vi "Read id.vi"(8 "error in (no error)":errorcluster, 11 "Motor in":refnum<class "Motor.lvclass">) -> (0 "error out":errorcluster, 2 "id":string, 3 "Motor out":refnum<class "Motor.lvclass">)   [LabVIEW 2018, in "Motor.lvclass"]
uses:
  Motor.lvclass
  Motor.lvclass/Motor.ctl
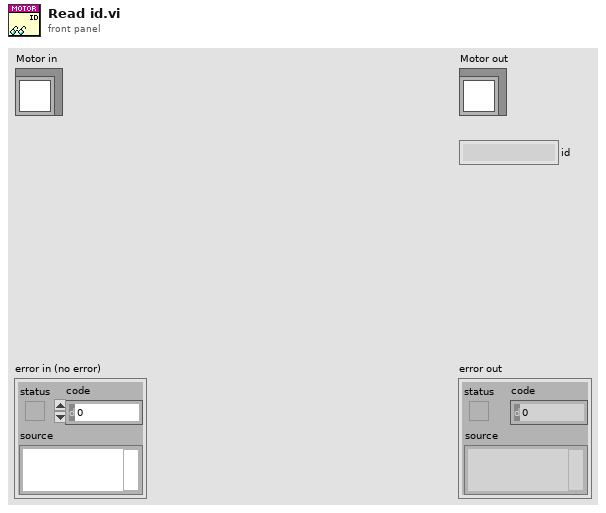
[diagram p1: front panel]
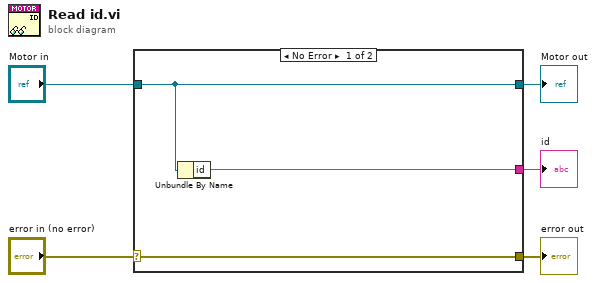
[diagram p0: block diagram]
diagram:
  n1 = case shown="No Error" "error in (no error)" {
    selector: "error in (no error)" -> [w8 w9]
    tunnel: [w8 w9] -> w4
    tunnel: [w7 w10] -> w2
    tunnel: "Motor in" -> [w7 w10]
    tunnel: [w6 _] -> w1
    frame No Error {
      n2 = Unbundle By Name(w7) -> ("id"=w6:string)
    }
    frame Error {
    }
  }
  "error out" <- w4
  "Motor out" <- w2
  "id" <- w1
